vi "TryUpdateDisplacementSample.vi"   [LabVIEW 2018]
uses:
  <vilib>/Platform/TimedLoop/XDataNode/timing_clust.ctl
  <vilib>/Platform/TimedLoop/XDataNode/nitl_modes.ctl
  <vilib>/Platform/TimedLoop/XDataNode/wakeup.ctl
  Telemetry/TelemetryDataTypes.ctl
  Telemetry/TelemetryUpdateModes.ctl
  Telemetry/TelemetryFields.ctl
  <vilib>/rvi/Emulation/niFpgaEmulationIsFPGAContextNoSignature.vi
  <vilib>/rvi/Emulation/niFpgaSctlEmulationGetInTimedLoop.vi
  <vilib>/rvi/errors/niFpgaSetErrorForExecOnDevCompSimple.vi
  <vilib>/rvi/eio/common/nirviEmuReportErrorAndStop.vi
  <vilib>/rvi/DataTransferAndStorage/Container/Common/niFpgaContainerGetUniqueNameForEmu.vi
  <vilib>/rvi/FIFO/Fifo_Resource/nirvififoEmulationSetSize.vi
  <vilib>/rvi/FIFO/Fifo_Resource/nirviFifoEmulationQueueMgr.vi
  <instcachedir>/0/nirviFifoEmulationQueueMgr_E5CAEC123FF24DC58D834DCA3CDAA9B5.lvgen/nirviFifoEmulationQueueMgr_E5CAEC123FF24DC58D834DCA3CDAA9B5_016.vi
  <vilib>/Utility/error.llb/Clear Errors.vi
  <vilib>/rvi/FIFO/Fifo_Resource/nirvififoEmulationCreateLock.vi
  <vilib>/rvi/Emulation/niFpgaProcessEmulError.vi
  <vilib>/rvi/FIFO/Fifo_Resource/nirvififoEmulationObtainLock.vi
  <vilib>/rvi/FIFO/Fifo_Resource/nirvififoEmulationReleaseLock.vi
  <vilib>/rvi/occurrence/nirviWaitOnOccurrenceBase.vi
  <vilib>/rvi/errors/nirviReportUnexpectedCaseInternalError.vi
  <vilib>/rvi/errors/nirviReportUnexpectedCaseInternalError (U32).vi
  <vilib>/rvi/Emulation/niFpgaEmulationReportErrorSimple.vi
  <vilib>/rvi/Emulation/niFpgaGetClockAttributes.vi
  <vilib>/rvi/Emulation/niFpgaCriticalErrorInLSC.vi
  <instcachedir>/0/nirviFifoEmulationQueueMgr_E5CAEC123FF24DC58D834DCA3CDAA9B5.lvgen/nirviFifoEmulationQueueMgr_E5CAEC123FF24DC58D834DCA3CDAA9B5_007.vi
  <vilib>/rvi/FIFO/Fifo_Resource/nirvififoEmulationDetermineInputValidOut.vi
  <vilib>/rvi/Memory/Memory_Emulation/niFpgaMemoryEmulationCacheClearOnFirstRun.vi
  <vilib>/rvi/Memory/Memory_Emulation/nirvimemoryEmulationManagerCache_MakeExclusive.vi
  <vilib>/rvi/Memory/Memory_Emulation/niFpgaMemoryEmulationValidateCache.vi
  <vilib>/rvi/Memory/Memory_Emulation/nirvimemoryEmulationManagerCache_InsertValue.vi
  <vilib>/rvi/Memory/Memory_Emulation/nirvimemoryEmulationManagerCache_ReleaseExclusive.vi
  <vilib>/rvi/Memory/Memory_Emulation/nirvimemoryEmulationManagerCache_GetValue.vi
  <vilib>/rvi/Memory/Memory_Emulation/nirvimemoryEmulationManagerCache_SetValue.vi
  <instcachedir>/0/nirviFifoEmulationQueueMgr_E5CAEC123FF24DC58D834DCA3CDAA9B5.lvgen/nirviFifoEmulationQueueMgr_E5CAEC123FF24DC58D834DCA3CDAA9B5_002.vi
  <vilib>/rvi/DataTransferAndStorage/Container/XNode/niFpgaContainer.xnode
  <vilib>/rvi/FIFO/Fifo_Resource/nirvififoEmulationRead.vi
  <vilib>/Platform/TimedLoop/XDataNode/XDataNode.xnode
  <vilib>/rvi/FIFO/Fifo_Resource/nirvififoEmulationWrite.vi
  <vilib>/rvi/DataTransferAndStorage/Register/Emulation/niFpgaRegisterEmulation.vi
  <vilib>/Platform/TimedLoop/XDataNode/XDNodeRunTimeDep.lvlib
types:
  T1 = cluster{"Timestamp":u64, "TxBytes":u64, "RxBytes":u64, "TxFrames":u64, "RxFrames":u64, "Sensor1Raw":i32, "Sensor2Raw":i32, "Sensor3Raw":i32, "Sensor4Raw":i32, "Sensor5Raw":i32, "Sensor6Raw":i32, "Sensor7Raw":i32, "Sensor8Raw":i32}
  T2 = typedef "TelemetryFields.ctl" = enum16{"None", "InclinometerTxBytes", "InclinometerRxBytes", "InclinometerTxFrames", "InclinometerRxFrames", "InclinometerErrorTimestamp", "InclinometerErrorCode", "InclinometerSampleTimestamp", "InclinometerAngleRaw", "DisplacementTxBytes", "DisplacementRxBytes", "DisplacementTxFrames", "DisplacementRxFrames", "DisplacementErrorTimestamp", "DisplacementErrorCode", "DisplacementSampleTimestamp", "DisplacementRaw1", "DisplacementRaw2", "DisplacementRaw3", "DisplacementRaw4", "DisplacementRaw5", "DisplacementRaw6", "DisplacementRaw7", "DisplacementRaw8", "AccelerometerSampleCount", "AccelerometerSampleTimestamp", "AccelerometerRaw1", "AccelerometerRaw2", "AccelerometerRaw3", "AccelerometerRaw4", "AccelerometerRaw5", "AccelerometerRaw6", "AccelerometerRaw7", "AccelerometerRaw8", "GyroTxBytes", "GyroRxBytes", "GyroTxFrames", "GyroRxFrames", "GyroErrorTimestamp", "GyroErrorCode", "GyroSampleTimestamp", "GyroRawX", "GyroRawY", "GyroRawZ", "GyroStatus", "GyroSequenceNumber", "GyroTemperature", "GyroBITTimestamp", "GyroBIT0", "GyroBIT1", "GyroBIT2", "GyroBIT3", "GyroBIT4", "GyroBIT5", "GyroBIT6", "GyroBIT7", "DigitalInputSampleCount", "DigitalInputTimestamp", "DigitalInputStates", "DigitalOutputSampleCount", "DigitalOutputTimestamp", "DigitalOutputStates", "PowerSupplySampleCount", "PowerSupplyTimestamp", "PowerSupplyStates", "Modbus1ErrorFlags", "Modbus1TxByteCount", "Modbus1TxFrameCount", "Modbus1RxByteCount", "Modbus1RxFrameCount", "Modbus2ErrorFlags", "Modbus2TxByteCount", "Modbus2TxFrameCount", "Modbus2RxByteCount", "Modbus2RxFrameCount", "Modbus3ErrorFlags", "Modbus3TxByteCount", "Modbus3TxFrameCount", "Modbus3RxByteCount", "Modbus3RxFrameCount", "Modbus4ErrorFlags", "Modbus4TxByteCount", "Modbus4TxFrameCount", "Modbus4RxByteCount", "Modbus4RxFrameCount"}
  T3 = typedef "TelemetryUpdateModes.ctl" = enum8{"=", "+", "-", "|"}
  T4 = typedef "TelemetryDataTypes.ctl" = enum8{"U8", "U16", "U32", "U64", "I8", "I16", "I32", "I64", "SGL"}
  T5 = typedef "XDNodeRunTimeDep.lvlib/timing_clust.ctl" = cluster{"Expected End [f-1]":u64, "Actual End [f-1]":u64, "Finished Late? [f-1]":bool, "Expected End [i-1]":u64, "Actual End [i-1]":u64, "Finished Late? [i-1]":bool, "Expected Start [i]":u64, "Actual Start [i]":u64, "Expected Start [f]":u64, "Actual Start [f]":u64, "Source Name":string, "Structure Name":string, "Period":i64, "Deadline":i64, "Offset":i64, "Start":i64, "Priority":i32, "Timeout":i32, "Mode":T6, "Wakeup Reason":T7, "Error":errorcluster, "Source Type":string, "Secondary Source Type":string, "Global End Time":u64, "Global Start Time":u64, "Frame Duration":u64, "Iteration Duration":u64, "Assigned CPU":i32, "I/O Scan Engine Mode":u32}
  T6 = typedef "XDNodeRunTimeDep.lvlib/nitl_modes.ctl" = enum32{"No Change", "Process missed periods, maintain original phase", "Discard missed periods, maintain original phase", "Process missed periods, ignore original phase", "Discard missed periods, ignore original phase"}
  T7 = typedef "XDNodeRunTimeDep.lvlib/wakeup.ctl" = enum32{"Normal", "Aborted", "Asynchronous wakeup", "Timing source error", "Timed loop error", "Timeout"}
  T8 = typedef "TelemetryUpdateData.ctl" = cluster{"DataType":T4, "Mode":T3, "Field":T2, "Data":u64}
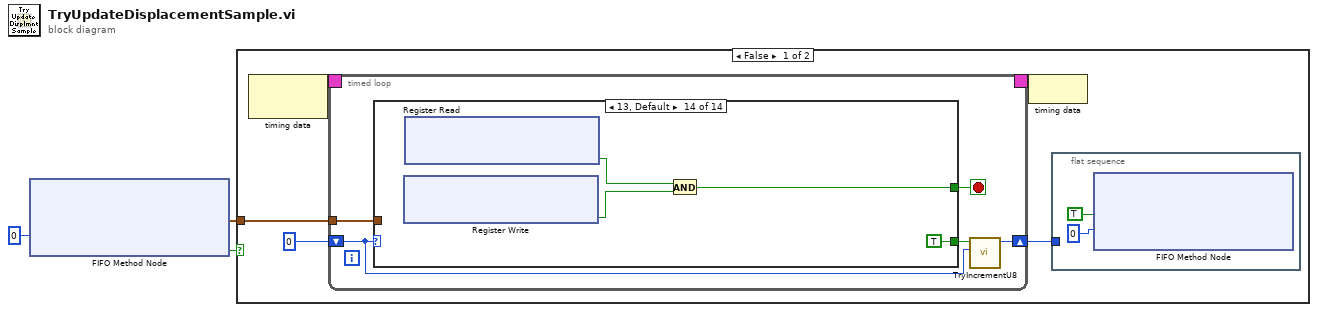
[diagram p0: block diagram]
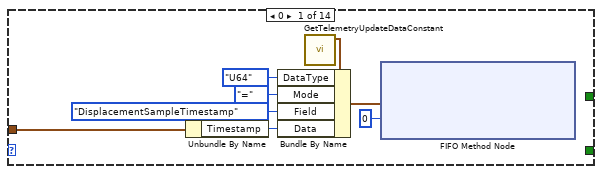
[diagram p2: hidden frame]
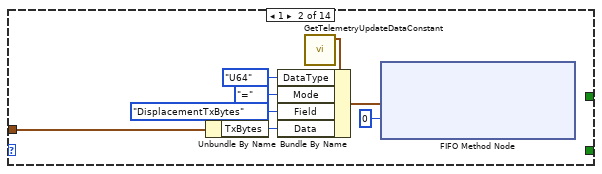
[diagram p3: hidden frame]
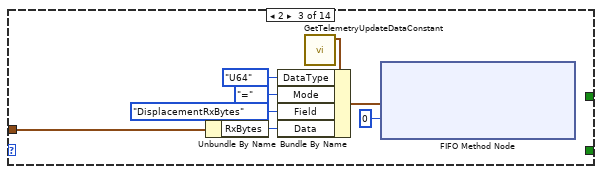
[diagram p4: hidden frame]
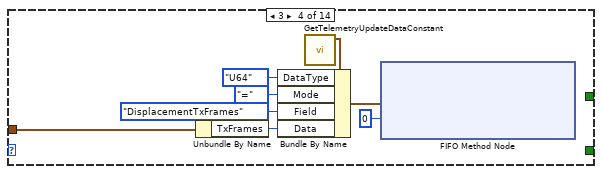
[diagram p5: hidden frame]
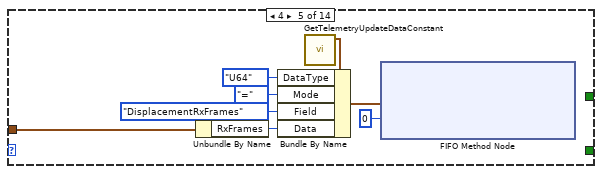
[diagram p6: hidden frame]
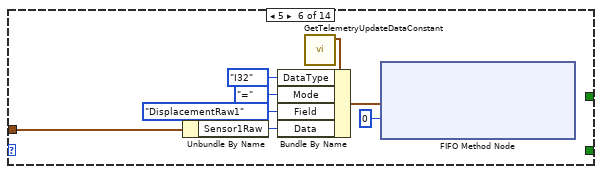
[diagram p7: hidden frame]
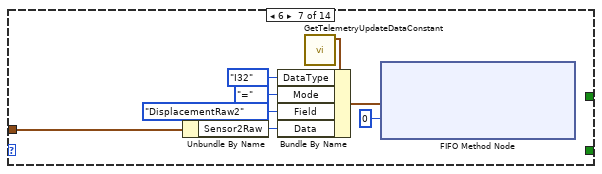
[diagram p8: hidden frame]
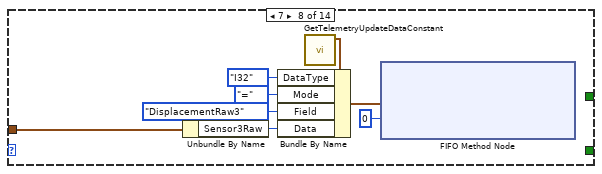
[diagram p9: hidden frame]
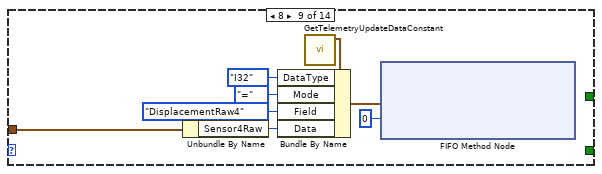
[diagram p10: hidden frame]
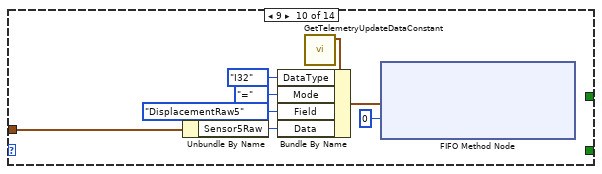
[diagram p11: hidden frame]
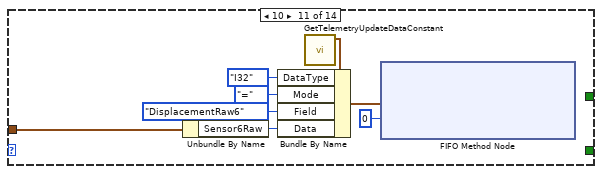
[diagram p12: hidden frame]
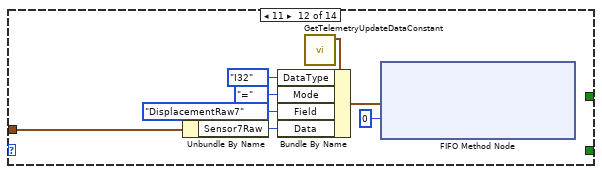
[diagram p13: hidden frame]
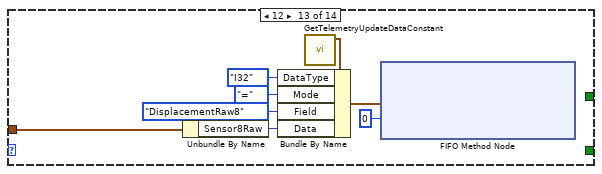
[diagram p14: hidden frame]
diagram:
  n1 = xnode ("FIFO Method Node")("Timeout"=0) -> ("Element"=w1:T1, "Timed Out?"=w2:bool)  [unwired: 1 in, 1 out]
  n2 = case shown="False" w2 {
    tunnel: w1 -> [w8 _]
    frame False {
      n3 = node-c288() -> (w7:T5)  [unwired: 1 in]
      n4 = timed-loop {
        tunnel: w8 -> [w13]
        timing: w7 -> [_]
        timing-out: [_] -> w6
        shift-right: [w11] -> w4
        shift-left: u8 0 -> [w10]
        stop <- w12 stop-if-true
        n5 = case shown="13, Default" w10 {
          tunnel: w13 -> [w14 w22 w30 w38 w46 w54 w62 w70 w78 w86 w94 w102 w110 _]
          tunnel: [_ _ _ _ _ _ _ _ _ _ _ _ _ w119] -> w12
          tunnel: [_ _ _ _ _ _ _ _ _ _ _ _ _ TRUE] -> w9
          frame 0 {
            n6 = Unbundle By Name(w14) -> ("Timestamp"=w20:u64)
            n7 = call "GetTelemetryUpdateDataConstant.vi"() -> ("TelemetryUpdateData"=w19:T8)  [unwired: 11 in]
            n8 = Bundle By Name(cluster=w19, "DataType"=TelemetryDataTypes."U64", "Mode"=TelemetryUpdateModes."=", "Field"=TelemetryFields."DisplacementSampleTimestamp" ("TelemetryFields"), "Data"=w20) -> (w16:T8)
            n9 = xnode ("FIFO Method Node")("Element"=w16, "Timeout"=0) -> ()  [unwired: 1 in, 2 out]
          }
          frame 1 {
            n10 = Unbundle By Name(w22) -> ("TxBytes"=w23:u64)
            n11 = call "GetTelemetryUpdateDataConstant.vi"() -> ("TelemetryUpdateData"=w24:T8)  [unwired: 11 in]
            n12 = Bundle By Name(cluster=w24, "DataType"=TelemetryDataTypes."U64", "Mode"=TelemetryUpdateModes."=", "Field"=TelemetryFields."DisplacementTxBytes", "Data"=w23) -> (w28:T8)
            n13 = xnode ("FIFO Method Node")("Element"=w28, "Timeout"=0) -> ()  [unwired: 1 in, 2 out]
          }
          frame 2 {
            n14 = Unbundle By Name(w30) -> ("RxBytes"=w37:u64)
            n15 = call "GetTelemetryUpdateDataConstant.vi"() -> ("TelemetryUpdateData"=w36:T8)  [unwired: 11 in]
            n16 = Bundle By Name(cluster=w36, "DataType"=TelemetryDataTypes."U64", "Mode"=TelemetryUpdateModes."=", "Field"=TelemetryFields."DisplacementRxBytes", "Data"=w37) -> (w32:T8)
            n17 = xnode ("FIFO Method Node")("Element"=w32, "Timeout"=0) -> ()  [unwired: 1 in, 2 out]
          }
          frame 3 {
            n18 = Unbundle By Name(w38) -> ("TxFrames"=w39:u64)
            n19 = call "GetTelemetryUpdateDataConstant.vi"() -> ("TelemetryUpdateData"=w40:T8)  [unwired: 11 in]
            n20 = Bundle By Name(cluster=w40, "DataType"=TelemetryDataTypes."U64", "Mode"=TelemetryUpdateModes."=", "Field"=TelemetryFields."DisplacementTxFrames", "Data"=w39) -> (w44:T8)
            n21 = xnode ("FIFO Method Node")("Element"=w44, "Timeout"=0) -> ()  [unwired: 1 in, 2 out]
          }
          frame 4 {
            n22 = Unbundle By Name(w46) -> ("RxFrames"=w53:u64)
            n23 = call "GetTelemetryUpdateDataConstant.vi"() -> ("TelemetryUpdateData"=w52:T8)  [unwired: 11 in]
            n24 = Bundle By Name(cluster=w52, "DataType"=TelemetryDataTypes."U64", "Mode"=TelemetryUpdateModes."=", "Field"=TelemetryFields."DisplacementRxFrames", "Data"=w53) -> (w48:T8)
            n25 = xnode ("FIFO Method Node")("Element"=w48, "Timeout"=0) -> ()  [unwired: 1 in, 2 out]
          }
          frame 5 {
            n26 = Unbundle By Name(w54) -> ("Sensor1Raw"=w55:i32)
            n27 = call "GetTelemetryUpdateDataConstant.vi"() -> ("TelemetryUpdateData"=w56:T8)  [unwired: 11 in]
            n28 = Bundle By Name(cluster=w56, "DataType"=TelemetryDataTypes."I32", "Mode"=TelemetryUpdateModes."=", "Field"=TelemetryFields."DisplacementRaw1" ("TelemetryFields"), "Data"=w55) -> (w59:T8)
            n29 = xnode ("FIFO Method Node")("Element"=w59, "Timeout"=0) -> ()  [unwired: 1 in, 2 out]
          }
          frame 6 {
            n30 = Unbundle By Name(w62) -> ("Sensor2Raw"=w68:i32)
            n31 = call "GetTelemetryUpdateDataConstant.vi"() -> ("TelemetryUpdateData"=w67:T8)  [unwired: 11 in]
            n32 = Bundle By Name(cluster=w67, "DataType"=TelemetryDataTypes."I32", "Mode"=TelemetryUpdateModes."=", "Field"=TelemetryFields."DisplacementRaw2" ("TelemetryFields"), "Data"=w68) -> (w64:T8)
            n33 = xnode ("FIFO Method Node")("Element"=w64, "Timeout"=0) -> ()  [unwired: 1 in, 2 out]
          }
          frame 7 {
            n34 = Unbundle By Name(w70) -> ("Sensor3Raw"=w71:i32)
            n35 = call "GetTelemetryUpdateDataConstant.vi"() -> ("TelemetryUpdateData"=w72:T8)  [unwired: 11 in]
            n36 = Bundle By Name(cluster=w72, "DataType"=TelemetryDataTypes."I32", "Mode"=TelemetryUpdateModes."=", "Field"=TelemetryFields."DisplacementRaw3" ("TelemetryFields"), "Data"=w71) -> (w75:T8)
            n37 = xnode ("FIFO Method Node")("Element"=w75, "Timeout"=0) -> ()  [unwired: 1 in, 2 out]
          }
          frame 8 {
            n38 = Unbundle By Name(w78) -> ("Sensor4Raw"=w84:i32)
            n39 = call "GetTelemetryUpdateDataConstant.vi"() -> ("TelemetryUpdateData"=w83:T8)  [unwired: 11 in]
            n40 = Bundle By Name(cluster=w83, "DataType"=TelemetryDataTypes."I32", "Mode"=TelemetryUpdateModes."=", "Field"=TelemetryFields."DisplacementRaw4" ("TelemetryFields"), "Data"=w84) -> (w80:T8)
            n41 = xnode ("FIFO Method Node")("Element"=w80, "Timeout"=0) -> ()  [unwired: 1 in, 2 out]
          }
          frame 9 {
            n42 = Unbundle By Name(w86) -> ("Sensor5Raw"=w87:i32)
            n43 = call "GetTelemetryUpdateDataConstant.vi"() -> ("TelemetryUpdateData"=w88:T8)  [unwired: 11 in]
            n44 = Bundle By Name(cluster=w88, "DataType"=TelemetryDataTypes."I32", "Mode"=TelemetryUpdateModes."=", "Field"=TelemetryFields."DisplacementRaw5" ("TelemetryFields"), "Data"=w87) -> (w91:T8)
            n45 = xnode ("FIFO Method Node")("Element"=w91, "Timeout"=0) -> ()  [unwired: 1 in, 2 out]
          }
          frame 10 {
            n46 = Unbundle By Name(w94) -> ("Sensor6Raw"=w100:i32)
            n47 = call "GetTelemetryUpdateDataConstant.vi"() -> ("TelemetryUpdateData"=w99:T8)  [unwired: 11 in]
            n48 = Bundle By Name(cluster=w99, "DataType"=TelemetryDataTypes."I32", "Mode"=TelemetryUpdateModes."=", "Field"=TelemetryFields."DisplacementRaw6" ("TelemetryFields"), "Data"=w100) -> (w96:T8)
            n49 = xnode ("FIFO Method Node")("Element"=w96, "Timeout"=0) -> ()  [unwired: 1 in, 2 out]
          }
          frame 11 {
            n50 = Unbundle By Name(w102) -> ("Sensor7Raw"=w103:i32)
            n51 = call "GetTelemetryUpdateDataConstant.vi"() -> ("TelemetryUpdateData"=w104:T8)  [unwired: 11 in]
            n52 = Bundle By Name(cluster=w104, "DataType"=TelemetryDataTypes."I32", "Mode"=TelemetryUpdateModes."=", "Field"=TelemetryFields."DisplacementRaw7" ("TelemetryFields"), "Data"=w103) -> (w107:T8)
            n53 = xnode ("FIFO Method Node")("Element"=w107, "Timeout"=0) -> ()  [unwired: 1 in, 2 out]
          }
          frame 12 {
            n54 = Unbundle By Name(w110) -> ("Sensor8Raw"=w116:i32)
            n55 = call "GetTelemetryUpdateDataConstant.vi"() -> ("TelemetryUpdateData"=w115:T8)  [unwired: 11 in]
            n56 = Bundle By Name(cluster=w115, "DataType"=TelemetryDataTypes."I32", "Mode"=TelemetryUpdateModes."=", "Field"=TelemetryFields."DisplacementRaw8" ("TelemetryFields"), "Data"=w116) -> (w112:T8)
            n57 = xnode ("FIFO Method Node")("Element"=w112, "Timeout"=0) -> ()  [unwired: 1 in, 2 out]
          }
          frame 13, Default {
            n58 = xnode "Register Write"() -> ("Data"=w121:bool)  [unwired: 1 in, 1 out]
            n59 = xnode ("Register Read")() -> ("Data"=w120:bool)  [unwired: 1 in, 1 out]
            n60 = And(x=w120, y=w121) -> (x .and. y?=w119:bool)
          }
        }
        n61 = call "TryIncrementU8.vi"("In"=w10, "DontInc"=w9) -> ("Out"=w11:u8)  [unwired: 9 in]
      }
      n62 = node-c288(w6) -> ()
      n63 = flat-sequence {
        tunnel: w4 -> [_]
        frame #0 {
          n64 = xnode ("FIFO Method Node")("Element"=TRUE, "Timeout"=0) -> ()  [unwired: 1 in, 2 out]
        }
      }
    }
    frame True {
    }
  }
